vi "ParseData.vi"(1 "input string":string) -> (0 "output cluster":T1)   [LabVIEW 2023]
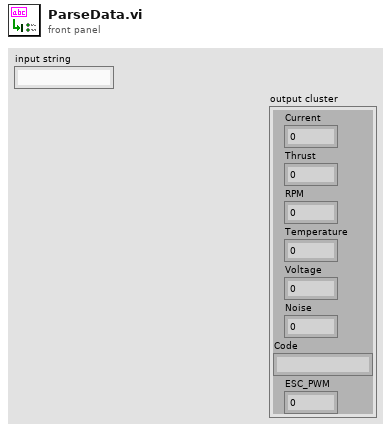
[diagram p1: front panel]
types:
  T1 = cluster{"Current":dbl, "Thrust":dbl, "RPM":dbl, "Temperature":dbl, "Voltage":dbl, "Noise":dbl, "Code":string, "ESC_PWM":i16}
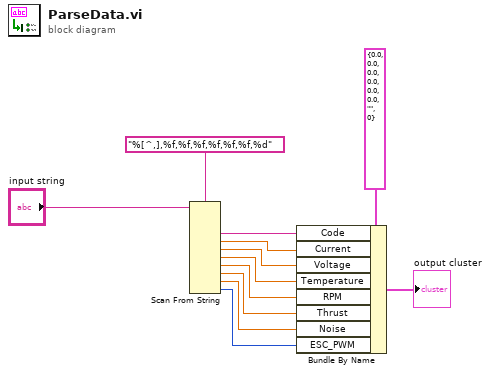
[diagram p0: block diagram]
diagram:
  n1 = Scan From String(format string="%[^,],%f,%f,%f,%f,%f,%f,%d", input string="input string") -> (output 1=w6:string, output 2=w7:dbl, output 3=w8:dbl, output 4=w9:dbl, output 5=w10:dbl, output 6=w11:dbl, output 7=w12:dbl, output 8=w3:i32)  [unwired: 10 in, 3 out]
  n2 = Bundle By Name(cluster=T1 {"Current"=0.0, "Thrust"=0.0, "RPM"=0.0, "Temperature"=0.0, "Voltage"=0.0, "Noise"=0.0, "Code"="", "ESC_PWM"=0} ("Data"), "Code"=w6, "Current"=w7, "Voltage"=w8, "Temperature"=w9, "RPM"=w10, "Thrust"=w11, "Noise"=w12, "ESC_PWM"=w3) -> (→"output cluster":T1)
